vi "CommandBST.vi"() -> ()   [LabVIEW 2013]
uses:
  <vilib>/Utility/file.llb/Write To Spreadsheet File (DBL).vi
panel:
  out "Time stamps":timestamp[](array[timestamp])
  in  "file path (dialog if empty)":path
  in  "Tab Control":enum32{"Page 1", "Page 2"}(tab)
  in  "K":u8
  in  "R":u8
  in  "-":u8
  in  "1":i32
  in  "N Data Size":u16
  in  "Boolean":bool
  out "Packet":dbl[](array[numeric])
  out "Array":u8[](array[numeric])
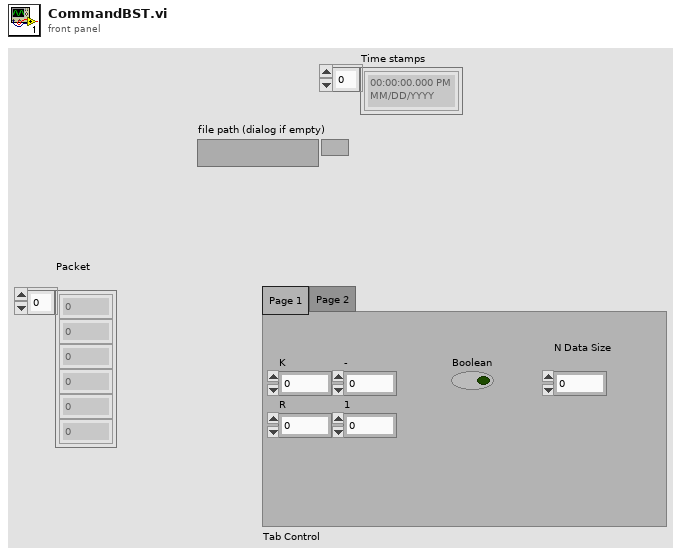
[diagram p1: front panel]
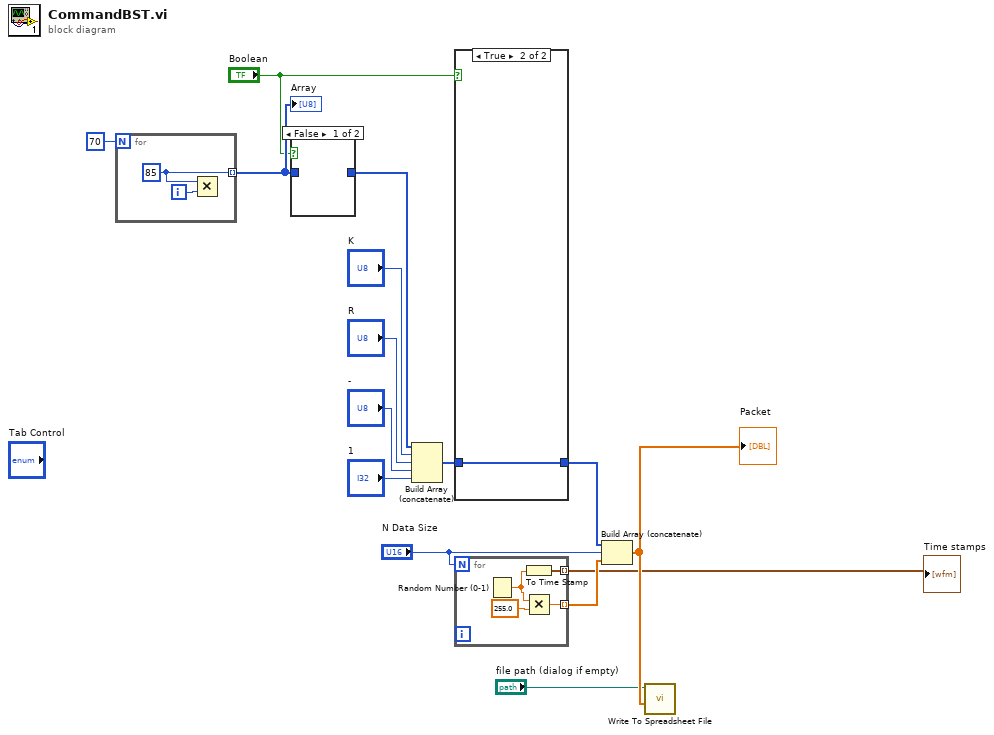
[diagram p0: block diagram]
diagram:
  n1 = for {
    N: 70 -> [_]
    tunnel: [w16] -> w14 mode=indexing
    i -> [w17]
    w16 = 85 ("x")
    n2 = Multiply(x=w16, y=w17) -> ()  [unwired: 1 out]
  }
  "Array" <- w14
  n3 = case shown="False" "Boolean" {
    tunnel: w14 -> [_ w18]
    tunnel: [_ w18] -> w8
    frame False {
    }
    frame True {
    }
  }
  n4 = Build Array (concatenate)(w8, "K", "R", "-", "1") -> (w4:i32[])
  n5 = case shown="True" "Boolean" {
    tunnel: [_ w19] -> w7
    tunnel: w4 -> [_ w19]
    frame False {
    }
    frame True {
    }
  }
  n6 = for {
    N: "N Data Size" -> [_]
    tunnel: [w22] -> w5 mode=indexing
    tunnel: [w20] -> w1 mode=indexing
    n7 = Random Number (0-1)() -> (number: 0 to 1=w21:dbl)
    n8 = To Time Stamp(1:w21) -> (0:w20:timestamp)
    n9 = Multiply(x=w21, y=255.0) -> (x*y=w22:dbl)
  }
  "Time stamps" <- w1
  n10 = Build Array (concatenate)(w7, "N Data Size", w5) -> (w3:dbl[])
  "Packet" <- w3
  n11 = call-poly <vilib>:"Write To Spreadsheet File.vi"("1D data"=w3, "file path (dialog if empty)"="file path (dialog if empty)") -> ()  [unwired: 6 in, 1 out]
